vi "E14_Nodos_de_Propiedad.vi"() -> ()   [LabVIEW 2026]
panel:
  out "Elapsed Time (s)":dbl
  out "Running":bool
  in  "stop":bool
  out "Alarma 01":string
  out "Alarma 02":string
  out "Waveform Chart":cluster{dbl, dbl, dbl}(graph)
  in  "Parametros":cluster{"Gancia K":dbl, "Uo":dbl}
  in  "Medición simulada":dbl(slide) scale=0.0..20.0
  out "Nivel de tanque":dbl(slide) scale=0.0..8.0
  # "Nivel en m^3"
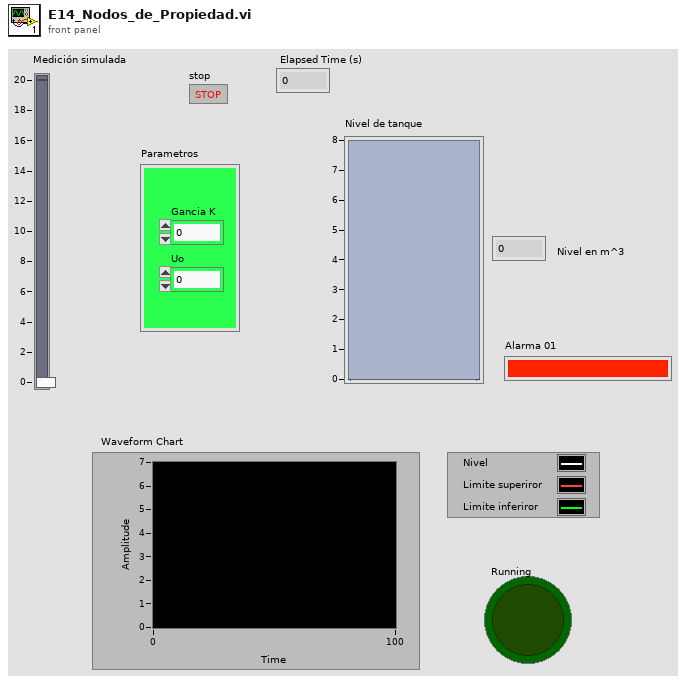
[diagram p1: front panel]
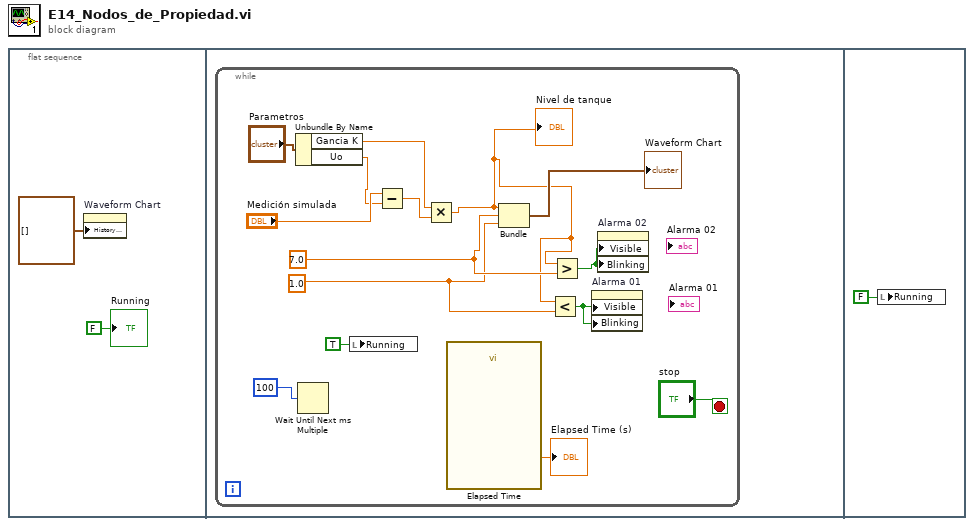
[diagram p0: block diagram]
diagram:
  n1 = flat-sequence {
    frame #0 {
      n2 = property on="Waveform Chart" class="WFChart (strict)"("History Data"=cluster{dbl, dbl, dbl}[] []) -> ()  [unwired: 2 in, 2 out]
      "Running" <- FALSE ("Running")
    }
    frame #1 {
      n3 = while {
        stop <- "stop" stop-if-true
        w7 = 1.0
        w9 = 7.0
        n4 = Unbundle By Name("Parametros") -> ("Gancia K"=w12:dbl, "Uo"=w14:dbl)
        n5 = Wait Until Next ms Multiple(millisecond multiple=100) -> ()  [unwired: 1 out]
        n6 = local write "Running"(TRUE ("Running")) -> ()
        n7 = Subtract(x="Medición simulada", y=w14) -> (x-y=w13:dbl)
        n8 = Multiply(x=w12, y=w13) -> (x*y=w8:dbl)
        "Nivel de tanque" <- w8
        n9 = call "Elapsed Time"() -> ("Elapsed Time (s)"=→"Elapsed Time (s)":dbl)  [unwired: 12 in, 7 out]
        n10 = Bundle(w8, w9, w7) -> (→"Waveform Chart":cluster{dbl, dbl, dbl})  [unwired: 1 in]
        n11 = Less?(x=w8, y=w7) -> (x < y?=w3:bool)
        n12 = Greater?(x=w8, y=w9) -> (0:w4:bool)
        n13 = property on="Alarma 01" class="Str"("Visible"=w3, "Blinking"=w3) -> ()  [unwired: 2 in, 2 out]
        n14 = property on="Alarma 02" class="Str"("Visible"=w4, "Blinking"=w4) -> ()  [unwired: 2 in, 2 out]
      }
    }
    frame #2 {
      n15 = local write "Running"(FALSE ("Running")) -> ()
    }
  }
